vi "Hardware-DCM-23XX-System.vi"(8 "error in (no error)":errorcluster, 9 "LoopCount":i32, 10 "LoopPeriod [usec]":u32, 11 "DSI Reference":refnum<class "DCM-DSI.lvclass">) -> (0 "error out":errorcluster, 3 "DSI Reference":refnum<class "DCM-DSI.lvclass">)   [LabVIEW 2016, in "DSI-RT.lvlib"]
uses:
  DSI-RT.lvlib
  Classes/DCM-DSI/DCM-DSI.lvclass
  <vilib>/Powertrain Controls/Device Drivers/DCM/Rev0/RT/DCM - RT.lvclass/DCM - RT.ctl
  <vilib>/Powertrain Controls/Device Drivers/DCM/Rev0/RT/Read dT (25n) [s].vi
  <vilib>/Powertrain Controls/Device Drivers/DCM/Rev0/RT/Write IO Lock.vi
  Classes/DCM-DSI/Read DCM Ref.vi
  Classes/DCM-DSI/Read DI-A Profiles.vi
  Classes/DCM-DSI/Read DI-B Profiles.vi
  Classes/DCM-DSI/Write LoopCount.vi
  Classes/DCM-DSI/Write dt.vi
  Classes/DCM-DSI/Write System State.vi
  Classes/DCM-DSI/Write HH Status.vi
  <vilib>/addons/Software Calibration Management/xSCM/CalPoint.xnode
  <vilib>/Powertrain Controls/Device Drivers/DCM/Rev0/RT/DCM - RT.lvclass
  <vilib>/addons/Software Calibration Management/xSCM/FaultPoint.xnode
  <vilib>/Powertrain Controls/Device Drivers/DCM/DI/RT/DCM - RT - DI.lvlib
  <vilib>/Powertrain Controls/Device Drivers/DCM/IRQ/RT/DCM - RT - IRQ.lvlib
  <vilib>/Powertrain Controls/Device Drivers/DCM/Tools/RT/DCM - RT - Tools.lvlib
  <vilib>/addons/Software Calibration Management/xSCM/ni_scm.dll
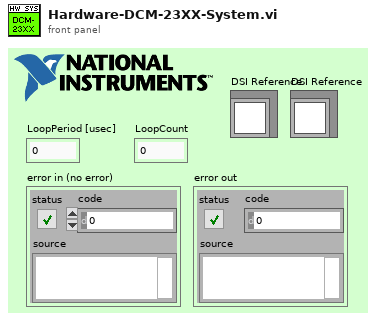
[diagram p1: front panel]
types:
  T1 = typedef "DCM - RT.lvclass/User LED.ctl" = enum16{"Off", "Yellow", "Green"}
  T2 = typedef "DCM - RT - DI.lvlib/Phase.ctl" = cluster{"Drive":T3, "Direction":bool, "Phase Step":T4, "Duration [s]":sgl, "Current High [A]":sgl, "Current Low [A]":sgl, "Voltage High [V]":sgl, "Voltage Low [V]":sgl, "Change":bool, "Current Control":T5, "Period [s]":sgl, "Pulse Width [s]":sgl, "Profile":u8, "Voltage Control":bool}
  T3 = typedef "DCM - FPGA.lvlib/DI - Drive State.ctl" = enum8{"Idle", "HV Current Control", "LV Current Control", "Back Boost", "Piezo Charge", "Piezo Discharge"}
  T4 = typedef "DCM - FPGA - DI.lvlib/Phase Step.ctl" = enum8{"Duration", "First Peak", "End of Cmd", "Branch", "2-Phase Duration"}
  T5 = typedef "DCM - FPGA - DI.lvlib/Control.ctl" = enum8{"Closed Loop", "Fixed Period", "Fixed On Pulse", "Fixed Off Pulse", "Open Loop", "Profile"}
  T6 = typedef "DCM - RT - Tools.lvlib/Knock Settings.ctl" = cluster{"Low Cutoff [Hz]":sgl, "High Cutoff [Hz]":sgl, "Threshold":sgl}
  T7 = typedef "Knock - RevA - RT.lvlib/Windows.ctl" = cluster{"Knock Start [CAD]":sgl, "Knock End [CAD]":sgl, "Reference Start [CAD]":sgl, "Reference End [CAD]":sgl}
  T8 = typedef "DCM - RT - IRQ.lvlib/IRQ Setup.ctl" = cluster{"Enable":bool, "Window Start [DBTDC]":sgl, "Window End [DBTDC]":sgl, "Location [DBTDC]":sgl, "TDC Offset [CAD]":sgl}
  T9 = typedef "EPTx - RevA - RT.lvlib/EPTxState.ctl" = cluster{"Sync Enable":bool, "Clear Errors":bool, "Sim Enable":bool, "Sim Speed [RPM]":sgl}
  T10 = typedef "DCM - FPGA.lvlib/Digital Channel.ctl" = enum8{"Unused", "User OS", "Diff IO 1", "Diff IO 2", "Diff IO 3", "Diff IO 4", "Diff IO 5", "Diff IO 6", "Diff IO 7", "Diff IO 8", "Aux 1", "Aux 2", "Aux 3", "Aux 4", "Aux 5", "Aux 6", "Aux 7", "Aux 8", "Aux 9", "Aux 10", "Aux 11", "Aux 12", "Aux 13", "Aux 14", "Aux 15", "Aux 16"}
  T11 = cluster{"Primary":T10, "Aux 1":T10, "Aux 2":T10, "Aux 3":T10, "Aux 4":T10}
  T12 = typedef "EPTx - RevA - RT.lvlib/EPTxFilters.ctl" = cluster{"Primary [s]":sgl, "Aux 1 [s]":sgl, "Aux 2 [s]":sgl, "Aux 3 [s]":sgl, "Aux 4 [s]":sgl}
  T13 = typedef "EPTx - RevA - RT.lvlib/EPTxData.ctl" = cluster{"Sync":bool, "CurrentCAD":sgl, "Speed [RPM]":sgl, "Config":bool, "Rcvg Primary":bool, "Stall":bool, "Overflow":bool, "Ratio Error":bool, "Pattern Error":bool, "Aux Warning":bool, "Watchdog Error":bool}
  T14 = typedef "DCM - RT.lvclass/System Settings.ctl" = cluster{"MPRD":bool, "IO Lock MPRD Disable":bool, "User LED 1":T1, "User LED 2":T1, "DI HS Fault Filter Time [s]":sgl, "Clamp Fault Filter Time [s]":sgl, "HH Shoot Through Time [s]":sgl, "HH ISeq Dur PS":T15, "HH Open Threshold [A]":sgl}
  T15 = typedef "DCM - RT - HH.lvlib/Duration Pre Scale.ctl" = u8
  T16 = typedef "DCM - RT.lvclass/Configuration.ctl" = cluster{"Configuration":T17, "Power Supply Enable":bool, "Boost Voltage [V]":sgl, "Inject Enable":bool, "DI Zener Enable":bool, "DI Zener Voltage [V]":sgl, "Pump Zener Enable":bool, "Pump Zener Voltage [V]":sgl, "Boost Clamp [V]":sgl}
  T17 = typedef "DCM - FPGA.lvlib/DI - Bank Configuration.ctl" = enum8{"Solenoid Unipolar 4", "Solenoid Unipolar 7 (Muxed)", "Solenoid Unipolar 8 (Muxed)", "Solenoid Bipolar 2", "Solenoid Bipolar 3 (Muxed)", "Piezo Unipolar 2", "Piezo Unipolar 3 (Muxed)", "Piezo Unipolar 4 (Muxed)", "Piezo Bipolar 2", "Piezo Bipolar 3 (Muxed)"}
  T18 = typedef "DCM - FPGA - Tools.lvlib/8 Channels.ctl" = cluster{"1":bool, "2":bool, "3":bool, "4":bool, "5":bool, "6":bool, "7":bool, "8":bool}
  T19 = typedef "DCM - RT - HH.lvlib/Mode.ctl" = enum16{"Off", "Lowside", "Highside", "PFI", "Full H", "3-Phase"}
  T20 = typedef "DCM - RT - HH.lvlib/ISeq.ctl" = cluster{"Upper [A]":sgl, "Lower [A]":sgl, "Duration [s]":sgl}
  T21 = cluster{"Mode":T19, "IO Lock State":bool, "Phase 1 FP":bool, "Fault Clear":bool, "ISeq":T20[]}[]
  T22 = typedef "DCM - RT.lvclass/Run State.ctl" = enum8{"Idle", "Warmup", "Ready To Inject", "Cool Down"}
  T23 = typedef "DCM - RT.lvclass/System State.ctl" = cluster{"System ADC":T24, "IO Lock":bool, "HH Mode Config Error":bool, "Fan Speed 1 [RPM]":sgl, "Fan Speed 2 [RPM]":sgl, "Firmware Major Rev":u16, "Firmware Minor Rev":u16, "Internal Fault":T25, "Fault Value":dbl}
  T24 = typedef "DCM - RT.lvclass/System ADC.ctl" = cluster{"AI 1 [V]":sgl, "AI 2 [V]":sgl, "AI 3 [V]":sgl, "AI 4 [V]":sgl, "AI 5 [V]":sgl, "AI 6 [V]":sgl, "AI 7 [V]":sgl, "AI 8 [V]":sgl, "AI 9 [V]":sgl, "AI 10 [V]":sgl, "AI 11 [V]":sgl, "AI 12 [V]":sgl, "Temp HH 1-6 [C]":sgl, "Temp HH 7-12 [C]":sgl, "Temp DI A [C]":sgl, "Temp DI Zener A [C]":sgl, "Temp DI B [C]":sgl, "Temp DI Zener B [C]":sgl, "Temp CPU [C]":sgl, "Temp Fan Intake [C]":sgl, "Temp Secondary A [C]":sgl, "Temp Primary A [C]":sgl, "Temp Boost B [C]":sgl, "Primary Range [V]":sgl, "Primary A1A2 [V]":sgl, "Primary A3A4 [V]":sgl, "Primary B3B4 [V]":sgl, "Primary B1B2 [V]":sgl, "Secondary A1A2 [V]":sgl, "Secondary A3A4 [V]":sgl, "Secondary B3B4 [V]":sgl, "Secondary B1B2 [V]":sgl, "Ext HV A [V]":sgl, "Ext HV B [V]":sgl, "FET Driver [V]":sgl, "Fan [V]":sgl, "Battery [V]":sgl, "DRVP [V]":sgl, "Key [V]":sgl, "DI Zener A [V]":sgl, "DI Zener B [V]":sgl, "Pump Zener A [V]":sgl, "Pump Zener B [V]":sgl, "MPRD [V]":sgl}
  T25 = typedef "DCM - RT.lvclass/Internal Fault.ctl" = enum32{"None", "Temp HH 1-6", "Temp HH 7-12", "Temp DI A", "Temp DI Zener A", "Temp DI B", "Temp DI Zener B", "Temp Intake", "Temp Primary A", "Temp Secondary A", "Temp Boost B", "Temp CPU", "Low Battery", "Inrush Protection", "A Run Enable", "B Run Enable"}
  T26 = typedef "DCM - FPGA.lvlib/DI - Faults.ctl" = cluster{"HV Fault":bool, "LV Fault":bool, "LS Fault":bool, "MUX Fault":bool, "Open Warning":bool}
  T27 = typedef "DCM - RT - HH.lvlib/Status.ctl" = cluster{"Current [A]":sgl, "Config Error":bool, "Short Fault":bool, "Open Fault":bool, "Period Min [A]":sgl, "Period Max [A]":sgl, "Period Avg [A]":sgl, "On Avg [A]":sgl}
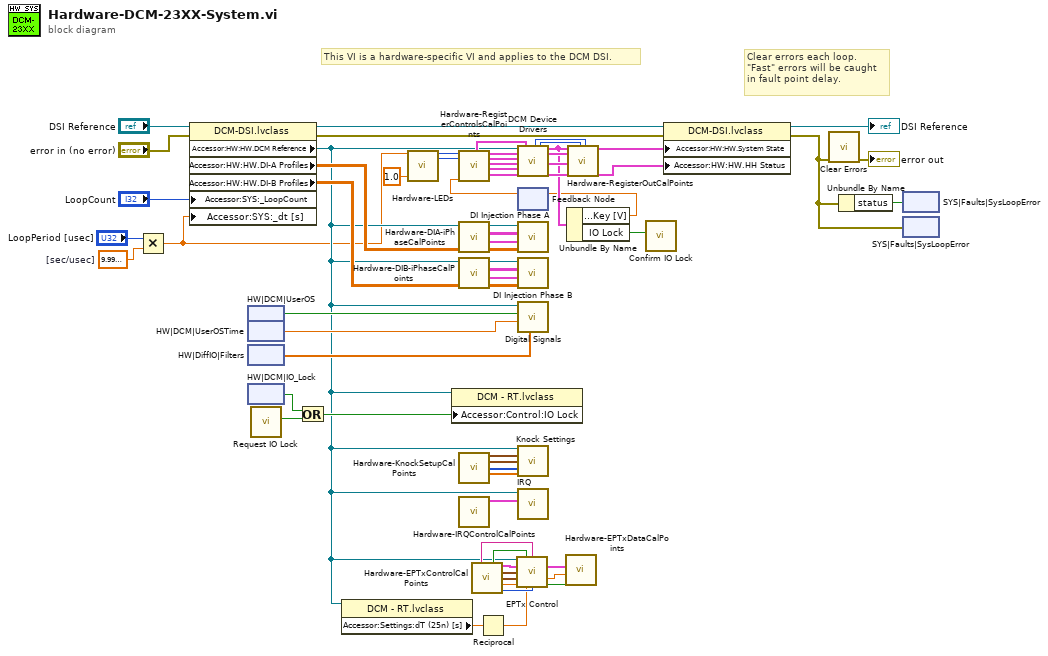
[diagram p0: block diagram]
diagram:
  w61 = sgl 1e-06  # [sec/usec]
  # "Clear errors each loop.\n\"Fast\" errors will be caught\nin fault point delay."
  # "This VI is a hardware-specific VI and applies to the DCM DSI."
  n1 = Multiply(x="LoopPeriod [usec]", y=w61) -> (x*y=w7:sgl)
  n2 = property class="DCM-DSI.lvclass"(reference="DSI Reference", error in="error in (no error)", "Accessor:SYS:_LoopCount"="LoopCount", "Accessor:SYS:_dt [s]"=w7) -> (reference out=w25:refnum<class "DCM-DSI.lvclass">, error out=w23:errorcluster, "Accessor:HW:HW.DCM Reference"=w10:refnum<class "DCM - RT.lvclass">, "Accessor:HW:HW.DI-A Profiles"=w22:sgl[][], "Accessor:HW:HW.DI-B Profiles"=w21:sgl[][])
  n3 = xnode "HW|DCM|UserOS"() -> ("Value"=w59:bool)
  n4 = xnode "HW|DCM|UserOSTime"() -> ("Value"=w58:sgl)
  n5 = xnode "HW|DiffIO|Filters"() -> ("Value"=w18:sgl[])
  n6 = xnode "HW|DCM|IO_Lock"() -> ("Value"=w15:bool)
  n7 = call <vilib>:"Request IO Lock.vi"() -> ("Request I/O Lock"=w13:bool)  [unwired: 11 in]
  n8 = Or(x=w15, y=w13) -> (x .or. y?=w14:bool)
  n9 = property class="DCM - RT.lvclass"(reference=w10) -> ("Accessor:Settings:dT (25n) [s]"=w9:sgl)  [unwired: 1 in, 2 out]
  n10 = call "Hardware-LEDs.vi"("LoopPeriod [sec]"=w7, "Activity Blink Rate [Hz]"=sgl 1.0 ("Desired Blink State Change [s]")) -> ("User LED 1"=w41:T1, "User LED 2"=w40:T1)  [unwired: 16 in]
  n11 = property class="DCM - RT.lvclass"(reference=w10, "Accessor:Control:IO Lock"=w14) -> ()  [unwired: 1 in, 2 out]
  n12 = call "Hardware-DIA-iPhaseCalPoints.vi"("A Profiles - Pulse Width [s]"=w22) -> ("A Profiles - Pulse Width [s]"=w52:sgl[][], "Pump-A Phase Arrays"=w51:T2[], "DI-A Phase Arrays"=w50:T2[][])  [unwired: 6 in]
  n13 = call "Hardware-DIB-iPhaseCalPoints.vi"("B Profiles - Pulse Width [s]"=w21) -> ("B Profiles - Pulse Width [s]"=w49:sgl[][], "Pump-B Phase Arrays"=w48:T2[], "DI-B Phase Arrays"=w47:T2[][])  [unwired: 6 in]
  n14 = call "Hardware-KnockSetupCalPoints.vi"() -> ("Knock Settings"=w57:T6, "Knock Windows"=w56:T7, "Knock Sensor"=w55:i32[], "Knock Offset [CAD]"=w54:sgl[])  [unwired: 12 in]
  n15 = call "Hardware-IRQControlCalPoints.vi"() -> ("IRQs"=w53:T8[])  [unwired: 11 in]
  n16 = call "Hardware-EPTxControlCalPoints.vi"() -> ("EPTx Settings File Path"=w38:string, "LoadEPTx Settings"=w37:bool, "EPTxState"=w36:T9, "EPTx Signal Select"=w35:T11, "EPTxFilters"=w34:T12, "StallSpeed [RPM]"=w33:sgl, "HistoryCAD"=w32:u8)  [unwired: 9 in]
  n17 = Reciprocal(x=w9) -> (1/x=w8:sgl)
  n18 = call <vilib>:"EPTx Control.vi"("DCM Reference"=w10, "Reload"=w37, "Settings File"=w38, "EPTxState"=w36, "EPTx Signal Select"=w35, "EPTxFilters"=w34, "Stall Speed [RPM]"=w33, "FPGA Frequency [Hz]"=w8, "History [CAD]"=w32) -> ("EPTxData"=w31:T13, "Max CAD"=w27:sgl, "Loading"=w28:bool)  [unwired: 3 in, 1 out]
  n19 = feedback #1() -> (w6:sgl)  [unwired: 1 in]
  n20 = call "Hardware-RegisterControlsCalPoints.vi"("User LED 1"=w41, "User LED 2"=w40, "Key [V]"=w6) -> ("System Settings"=w60:T14, "A Configuration"=w46:T16, "A Fault Clear"=w45:T18, "B Configuration"=w44:T16, "B Fault Clear"=w43:T18, "HW|HH|Config"=w42:T21)  [unwired: 11 in]
  n21 = call-dynamic "DCM Device Drivers.vi"("DCM Reference"=w10, "A Configuration"=w46, "A Fault Clear"=w45, "B Configuration"=w44, "B Fault Clear"=w43, "HH Config"=w42, "System Settings"=w60) -> ("A Run State"=w4:T22, "B Run State"=w3:T22, "System State"=w12:T23, "A DI Faults"=w30:T26[], "B DI Faults"=w29:T26[], "HH Status"=w19:T27[])  [unwired: 4 in, 3 out]
  n22 = call <vilib>:"DI Injection Phase A.vi"("Profile - Pulse Width [s]"=w52, "A Pump Phase Array"=w51, "A Phase Arrays"=w50, "DCM Reference"=w10) -> ()  [unwired: 8 in]
  n23 = call <vilib>:"DI Injection Phase B.vi"("Profile - Pulse Width [s]"=w49, "B Pump Phase Arrays"=w48, "B Phase Arrays"=w47, "DCM Reference"=w10) -> ()  [unwired: 8 in]
  n24 = call <vilib>:"Digital Signals.vi"("Diff IO Filters [s]"=w18, "User OS Time [s]"=w58, "User OS"=w59, "DCM Reference"=w10) -> ()  [unwired: 8 in]
  n25 = call <vilib>:"Knock Settings.vi"("DCM Reference"=w10, "Knock Settings"=w57, "Knock Windows"=w56, "Knock Sensor"=w55, "Knock Offset [CAD]"=w54) -> ()  [unwired: 11 in]
  n26 = call <vilib>:"IRQ.vi"("IRQs"=w53, "DCM Reference"=w10) -> ()  [unwired: 10 in]
  n27 = call "Hardware-EPTxDataCalPoints.vi"("Loading"=w28, "Max CAD"=w27, "EPTxData"=w31) -> ()  [unwired: 9 in]
  n28 = Unbundle By Name(w12) -> ("System ADC.Key [V]"=w5:sgl, "IO Lock"=w11:bool)
  n29 = feedback-in #1(w5) -> ()
  n30 = call "Hardware-RegisterOutCalPoints.vi"("System State"=w12, "DI-A Faults"=w30, "DI-B Faults"=w29, "HH Status"=w19, "B Run State"=w3, "A Run State"=w4) -> ()  [unwired: 14 in]
  n31 = call <vilib>:"Confirm IO Lock.vi"("Confirm I/O Locked"=w11) -> ()  [unwired: 11 in]
  n32 = property class="DCM-DSI.lvclass"(reference=w25, error in=w23, "Accessor:HW:HW.System State"=w12, "Accessor:HW:HW.HH Status"=w19) -> (reference out=→"DSI Reference":refnum<class "DCM-DSI.lvclass">, error out=w1:errorcluster)
  n33 = call <vilib>:"Clear Errors.vi"("error in (no error)"=w1) -> ("error out"=→"error out":errorcluster)  [unwired: 5 in, 1 out]
  n34 = Unbundle By Name(w1) -> ("status"=w16:bool)
  n35 = xnode "SYS|Faults|SysLoopError"("Fault"=w16) -> ()
  n36 = xnode "SYS|Faults|SysLoopError"("Value"=w1) -> ()
